vi "DHE_GetReadOverhead.vi"(9 "overhead string":string, 10 "Timing":T1 {"DET_READ_TIME" format="%.2f"; "known_overhead" format="%.2f"; "ShiftRow" format="%.2f"; "SkipRow" format="%.2f"; "SkipPixel" format="%.2f"; "PixelTime" format="%.2f"}) -> (1 "overhead":dbl)   [LabVIEW 2016]
uses:
  Common/public/vis/CMN_TimingInfo.ctl
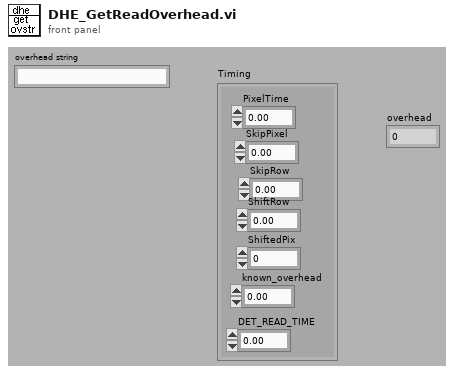
[diagram p1: front panel]
types:
  T1 = typedef "CMN_TimingInfo.ctl" = cluster{"PixelTime":sgl, "SkipPixel":sgl, "SkipRow":sgl, "ShiftRow":sgl, "ShiftedPix":u16, "known_overhead":sgl, "DET_READ_TIME":sgl}
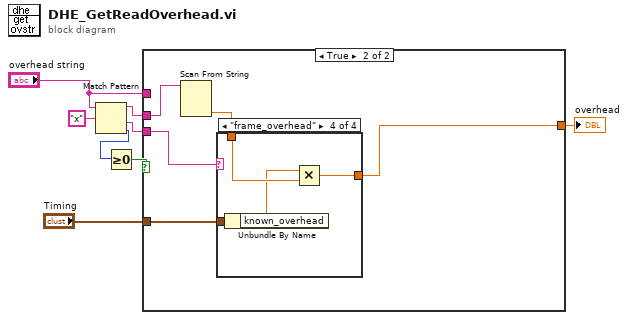
[diagram p0: block diagram]
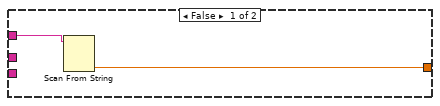
[diagram p2: hidden frame]
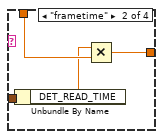
[diagram p4: hidden frame]
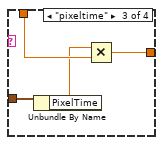
[diagram p5: hidden frame]
diagram:
  n1 = Match Pattern(string="overhead string", regular expression="x") -> (before substring=w4:string, after substring=w5:string, offset past match=w7:i32)  [unwired: 2 out]
  n2 = Greater Or Equal To 0?(x=w7) -> (x >= 0?=w6:bool)
  n3 = case shown="True" w6 {
    tunnel: "overhead string" -> [w10 _]
    tunnel: [w9 w12] -> w2
    tunnel: w5 -> [_ w14]
    tunnel: w4 -> [_ w15]
    tunnel: "Timing" -> [_ w11]
    frame False {
      n4 = Scan From String(input string=w10) -> (output 1=w9:dbl)  [unwired: 3 in, 4 out]
    }
    frame True {
      n5 = Scan From String(input string=w15) -> (output 1=w13:dbl)  [unwired: 3 in, 4 out]
      n6 = case shown="\"frame_overhead\"" w14 {
        tunnel: w13 -> [w16 w20 w24 w28]
        tunnel: [w16 w19 w23 w27] -> w12
        tunnel: w11 -> [_ w18 w22 w26]
        frame Default {
        }
        frame "frametime" {
          n7 = Unbundle By Name(w18) -> ("DET_READ_TIME"=w17:sgl)
          n8 = Multiply(x=w17, y=w20) -> (x*y=w19:dbl)
        }
        frame "pixeltime" {
          n9 = Unbundle By Name(w22) -> ("PixelTime"=w21:sgl)
          n10 = Multiply(x=w21, y=w24) -> (x*y=w23:dbl)
        }
        frame "frame_overhead" {
          n11 = Unbundle By Name(w26) -> ("known_overhead"=w25:sgl)
          n12 = Multiply(x=w25, y=w28) -> (x*y=w27:dbl)
        }
      }
    }
  }
  "overhead" <- w2
